vi "TreeNode Begin Timestamped Segment.vi"(8 "error in (no error)":errorcluster, 10 "Initial data":refnum<data-value>, 11 "TreeNode DVR in":refnum<data-value>) -> (0 "error out":errorcluster, 3 "TreeNode DVR out":refnum<data-value>)   [LabVIEW 2015, in "MDSplus.lvlib"]
doc: "Begin a new data segment."
uses:
  <vilib>/MDSplus/Library/MDSplus.lvlib
  <vilib>/MDSplus/Classes/Data_Class/TreeNode_Class/TreeNode.lvclass
  <vilib>/MDSplus/Classes/Data_Class/Array_Class/Array.lvclass
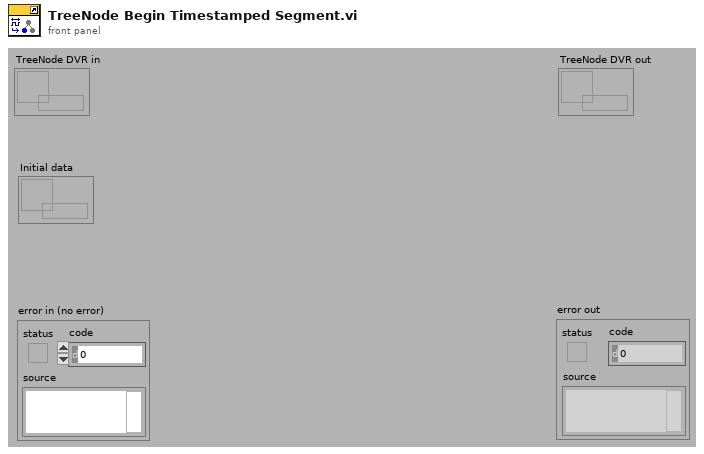
[diagram p1: front panel]
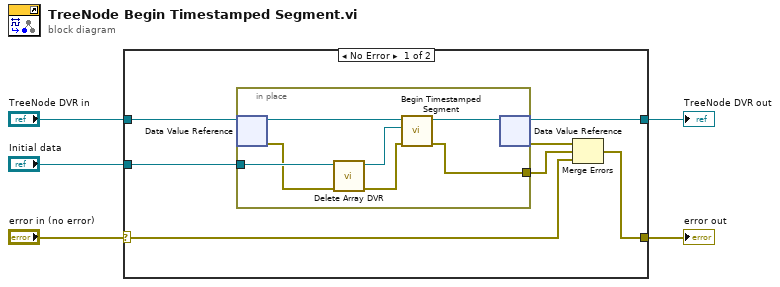
[diagram p0: block diagram]
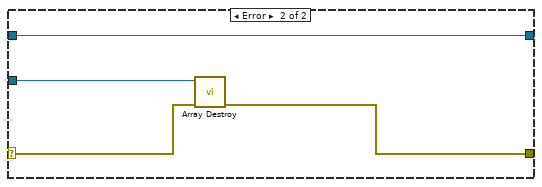
[diagram p2: hidden frame]
diagram:
  n1 = case shown="No Error" "error in (no error)" {
    selector: "error in (no error)" -> [w8 w22]
    tunnel: [w7 w20] -> w5
    tunnel: [w6 w21] -> w3
    tunnel: "Initial data" -> [w12 w23]
    tunnel: "TreeNode DVR in" -> [w11 w21]
    frame No Error {
      n2 = in-place {
        in-place-border: w12 -> [w19]
        in-place-border: [w17] -> w9
        n3 = in-place-dvr #1(w11) -> (w15:refnum<class "TreeNode.lvclass">, w18:errorcluster)
        n4 = call <vilib>:"Delete Array DVR.vi"("error in (no error)"=w18, "Array DVR in"=w19) -> ("error out"=w13:errorcluster, "Array out"=w14:refnum<class "Array.lvclass">)  [unwired: 8 in]
        n5 = call-dynamic "Begin Timestamped Segment.vi"("error in (no error)"=w13, "Initial data"=w14, "TreeNode in"=w15) -> ("error out"=w17:errorcluster, "TreeNode out"=w16:refnum<class "TreeNode.lvclass">)  [unwired: 7 in]
        n6 = in-place-dvr #1(w16) -> (w6:refnum<data-value>, w10:errorcluster)
      }
      n7 = Merge Errors(w10, w9, w8) -> (w7:errorcluster)
    }
    frame Error {
      n8 = call <vilib>:"Array Destroy.vi"("error in (no error)"=w22, "Array DVR in"=w23) -> ("error out"=w20:errorcluster)  [unwired: 9 in]
    }
  }
  "error out" <- w5
  "TreeNode DVR out" <- w3
